vi "02arma_panel.vi"(3 "EE 492":T1, 5 "Analogicas":dbl[](array[numeric])) -> (0 "Meds_17-32":string caption="MEDICIONES: 17-32", 1 "An. array":string[](array[string]), 2 "Meds_1-16":string caption="MEDICIONES: 1-16")   [LabVIEW 2010]
panel:
  in  "cantmedic":i32=32
  in  "Med_nom":string[](array[string])
  in  "Med_unid":string[](array[string])
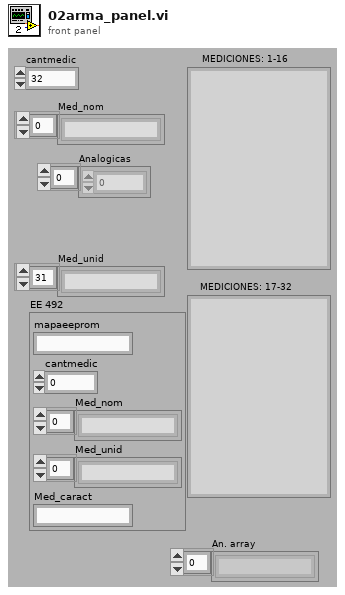
[diagram p1: front panel]
types:
  T1 = cluster{"mapaeeprom":string, "cantmedic":u8, "Med_nom":string[], "Med_unid":string[], "Med_caract":string}
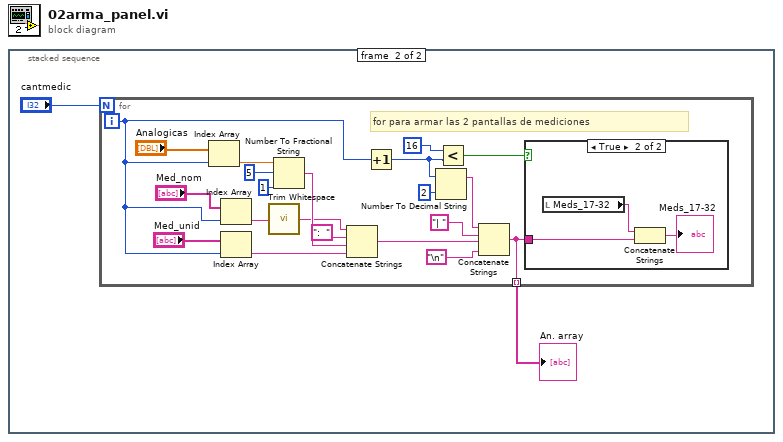
[diagram p0: block diagram]
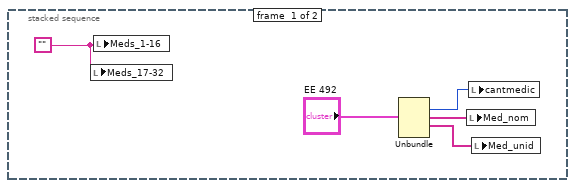
[diagram p2: hidden frame]
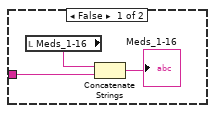
[diagram p3: hidden frame]
diagram:
  n1 = stacked-sequence {
    frame #0 {
      w5 = ""
      n2 = local write "Meds_17-32"(w5) -> ()
      n3 = local write "Meds_1-16"(w5) -> ()
      n4 = Unbundle("EE 492") -> ("cantmedic"=w1:u8, "Med_nom"=w2:string[], "Med_unid"=w3:string[])  [unwired: 2 out]
      n5 = local write "Med_nom"(w2) -> ()
      n6 = local write "cantmedic"(w1) -> ()
      n7 = local write "Med_unid"(w3) -> ()
    }
    frame #1 {
      n8 = for {
        N: "cantmedic" -> [_]
        tunnel: [w10] -> w6 mode=indexing
        i -> [w13]
        # "for para armar las 2 pantallas de mediciones"
        n9 = Index Array(array="Analogicas", index=w13) -> (element=w12:dbl)
        n10 = Index Array(array="Med_nom", index=w13) -> (element=w9:string)
        n11 = Index Array(array="Med_unid", index=w13) -> (element=w27:string)
        n12 = call <vilib>:"Trim Whitespace.vi"("string"=w9) -> ("trimmed string"=w8:string)  [unwired: 1 in]
        n13 = Number To Fractional String(number=w12, width (-)=i16 5, precision (6)=i16 1) -> (F-format string=w24:string)  [unwired: 1 out]
        n14 = Concatenate Strings(w8, ":  " ("Substring"), w24, w27) -> (w14:string)
        n15 = Increment(x=w13) -> (x+1=w18:i32)
        n16 = Number To Decimal String(number=w18, width (-)=i16 2) -> (decimal integer string=w15:string)
        n17 = Less?(x=16, y=w18) -> (x < y?=w20:bool)
        n18 = Concatenate Strings(w15, "| " ("string"), w14, "\n" ("string")) -> (w10:string)
        n19 = case shown="True" w20 {
          tunnel: w10 -> [w31 w32]
          frame False {
            n20 = local read "Meds_1-16"() -> (w30:string)
            n21 = Concatenate Strings(w30, w31) -> (→"Meds_1-16":string)
          }
          frame True {
            n22 = local read "Meds_17-32"() -> (w34:string)
            n23 = Concatenate Strings(w34, w32) -> (→"Meds_17-32":string)
          }
        }
      }
      "An. array" <- w6
    }
  }
